vi "In Aux Port.vi"(10 "state":i32, 11 "port":i32) -> (2 "state out":i32, 3 "function return":u32)   [LabVIEW 2018, in "Copy of Andor SDK.lvlib"]
doc: "EXPNETTYPE unsigned int WINAPI InAuxPort(int port, int * state);"
uses:
  Copy of Andor SDK.lvlib
  <userlib>/Andor SDK/ATMCD32D.dll
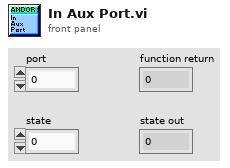
[diagram p1: front panel]
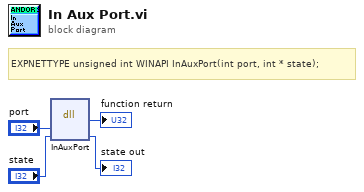
[diagram p0: block diagram]
diagram:
  # "EXPNETTYPE unsigned int WINAPI InAuxPort(int port, int * state);"
  n1 = dll-call lib="C:/Program Files (x86)/National Instruments/LabVIEW 2018/user.lib/Andor SDK/ATMCD32D.*" fn="InAuxPort"("port"="port", "state"="state") -> (→"function return":u32, "state"=→"state out":i32)  [unwired: 4 in, 2 out]
